vi "LEP_RV_WriteAllObjectsToXML.vi"(2 "error in":errorcluster, 3 "Data value reference for\nLabVIEW.map file's lines array":refnum<data-value>, 4 "XML File Refnum":refnum<file>) -> (0 "error out":errorcluster, 1 "Array with objects' names":string[](array[string]))   [LabVIEW 2011]
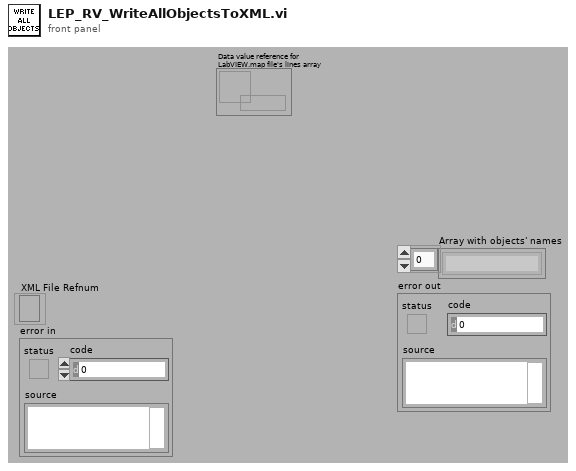
[diagram p1: front panel]
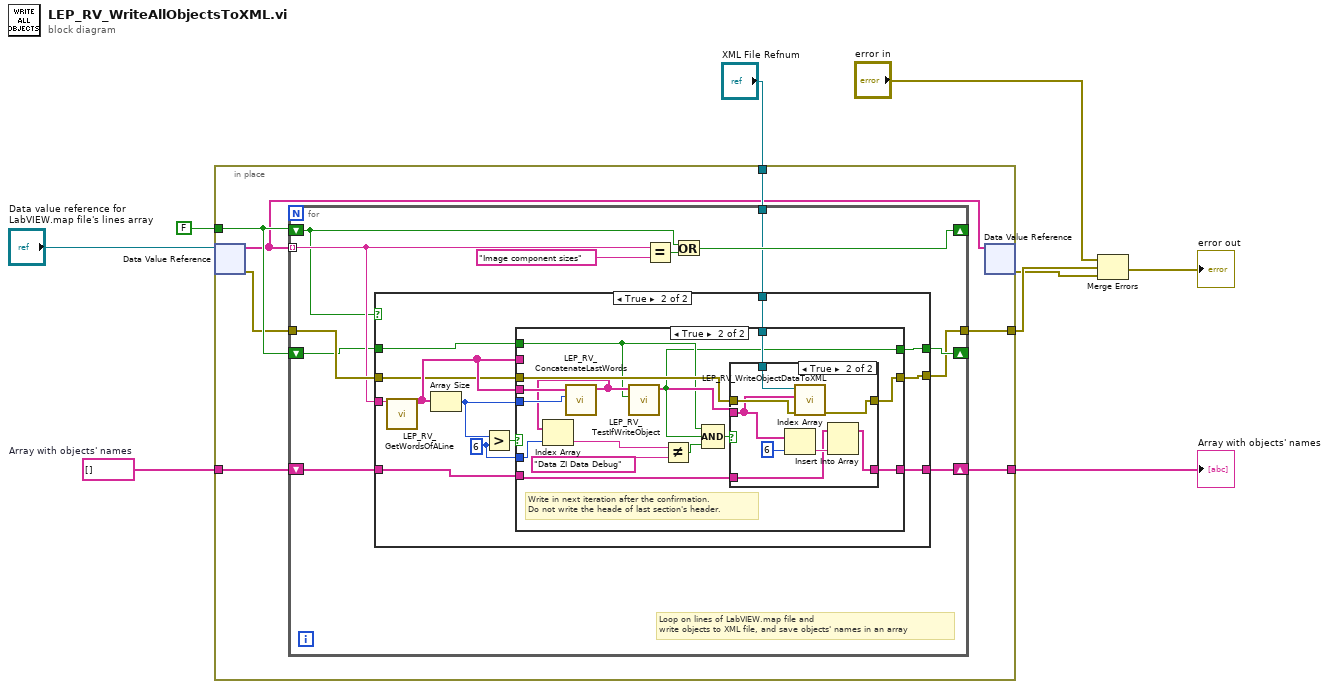
[diagram p0: block diagram]
diagram:
  w9 = string[] []  # Array with objects' names
  n1 = in-place {
    in-place-border: w9 -> [w16]
    in-place-border: [w15] -> w8
    in-place-border: FALSE -> [w14]
    in-place-border: [w13] -> w3
    in-place-border: "XML File Refnum" -> [w12]
    n2 = in-place-dvr #1("Data value reference for\nLabVIEW.map file's lines array") -> (w10:string[], w11:errorcluster)
    n3 = for {
      tunnel: w10 -> [w24] mode=indexing
      shift-right: [w26] -> _
      shift-left: w14 -> [w20]
      tunnel: w11 -> [w25]
      shift-right: [w21] -> w15
      shift-left: w16 -> [w23]
      tunnel: w12 -> [w22]
      shift-right: [w19] -> _
      shift-left: w14 -> [w18]
      tunnel: [w17] -> w13
      # "Loop on lines of LabVIEW.map file and \nwrite objects to XML file, and save objects' names in an array"
      n4 = case shown="True" w20 {
        tunnel: w24 -> [_ w40]
        tunnel: [w31 w39] -> w17
        tunnel: w25 -> [w31 w38]
        tunnel: w23 -> [w30 w37]
        tunnel: [w30 w36] -> w21
        tunnel: w22 -> [_ w35]
        tunnel: w18 -> [w29 w34]
        tunnel: [w29 w33] -> w19
        frame False {
        }
        frame True {
          w32 = 6 ("y")
          n5 = call "LEP_RV_GetWordsOfALine.vi"("Initial String"=w40) -> ("Array containing the words (tokens) of a string"=w41:string[])  [unwired: 9 in, 1 out]
          n6 = Array Size(array=w41) -> (size(s)=w42:i32)
          n7 = Greater?(x=w42, y=w32) -> (0:w43:bool)
          n8 = case shown="True" w43 {
            tunnel: w42 -> [_ w60]
            tunnel: w41 -> [_ _]
            tunnel: w41 -> [_ w61]
            tunnel: [w46 w59] -> w39
            tunnel: w38 -> [w46 w58]
            tunnel: w37 -> [w45 w47]
            tunnel: [w45 w57] -> w36
            tunnel: w35 -> [_ w56]
            tunnel: w34 -> [w44 w51]
            tunnel: [w44 w50] -> w33
            tunnel: w32 -> [_ w48]
            frame False {
            }
            frame True {
              # "Write in next iteration after the confirmation. \nDo not write the heade of last section's header."
              n9 = call "LEP_RV_ConcatenateLastWords.vi"("Initial array length"=w60, "Inittial array"=w61) -> ("Array containing exactly 7 words"=w53:string[])  [unwired: 9 in]
              n10 = Index Array(array=w53, index=w48) -> (element=w55:string)
              n11 = call "LEP_RV_TestIfWriteObject.vi"("Old decision"=w51, "Array of object's elements"=w53) -> ("Write ?"=w50:bool)  [unwired: 9 in]
              n12 = Not Equal?(x=w55, y="Data ZI Data Debug") -> (x != y?=w49:bool)
              n13 = Compound Arithmetic op=AND(w51, w50, w49) -> (w52:bool)
              n14 = case shown="True" w52 {
                tunnel: [w63 w70] -> w59
                tunnel: w58 -> [w63 w71]
                tunnel: w53 -> [_ w69]
                tunnel: w47 -> [w62 w66]
                tunnel: [w62 w65] -> w57
                tunnel: w56 -> [_ w64]
                frame False {
                }
                frame True {
                  n15 = Index Array(array=w69, index=6) -> (element=w67:string)
                  n16 = call "LEP_RV_WriteObjectDataToXML.vi"("error in"=w71, "Object elements array"=w69, "XMl file refnum"=w64) -> ("error out"=w70:errorcluster)  [unwired: 8 in]
                  n17 = Insert Into Array(array=w66, new element=w67) -> (w65:string[])  [unwired: 1 in]
                }
              }
            }
          }
        }
      }
      n18 = Equal?(x=w24, y="Image component sizes") -> (x = y?=w28:bool)
      n19 = Or(x=w20, y=w28) -> (x .or. y?=w26:bool)
    }
    n20 = in-place-dvr #1(w10) -> (w2:errorcluster)  [unwired: 1 out]
  }
  "Array with objects' names" <- w8
  n21 = Merge Errors("error in", w3, w2) -> (→"error out":errorcluster)
